vi "Create SubVI.vi"(8 "error in (no error)":errorcluster, 10 "Path":path, 11 "Diagram in":refnum<vi>) -> (0 "error out":errorcluster, 3 "subVI refnum":refnum<vi>)   [LabVIEW 2019, in "gRPC Template Creation Utility.lvlib"]
uses:
  <vilib>/Utility/miscctls.llb/LVPointTypeDef.ctl
  gRPC Template Creation Utility.lvlib
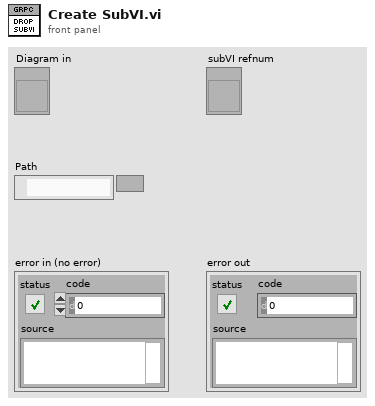
[diagram p1: front panel]
types:
  T1 = typedef "LVPointTypeDef.ctl" = cluster{"Horizontal":i16, "Vertical":i16}
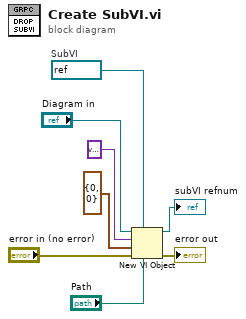
[diagram p0: block diagram]
diagram:
  w3 = refnum<vi> refnum  # SubVI
  n1 = New VI Object(vi object class=w3, owner refnum="Diagram in", style=variant, position/next to=T1 {"Horizontal"=0, "Vertical"=0} ("location"), 6:"Path", 8:"error in (no error)") -> (object refnum=→"subVI refnum":refnum<vi>, 0:→"error out":errorcluster)  [unwired: 2 in]
